vi "Periodic Tasks.vi"(8 "error in":errorcluster) -> ()   [LabVIEW 2023]
doc: "This VI runs in parallel to other tasks. It can contain as many user-defined periodic loops as you need. These can carry out PID or other sorts of timed response."
uses:
  <vilib>/Rock Robotics/WPI/Utilities/WPI_GetSetVariantRefNum.vi
  Robot Global Data.vi
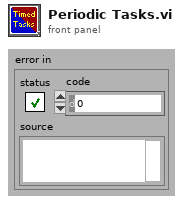
[diagram p1: front panel]
types:
  T1 = typedef "WPI_JoystickDevRef.ctl" = cluster{"Device":T2}
  T2 = typedef "WPI_JoystickDeviceEnum.ctl" = enum16{"USB 0", "USB 1", "USB 2", "USB 3", "USB 4", "USB 5"}
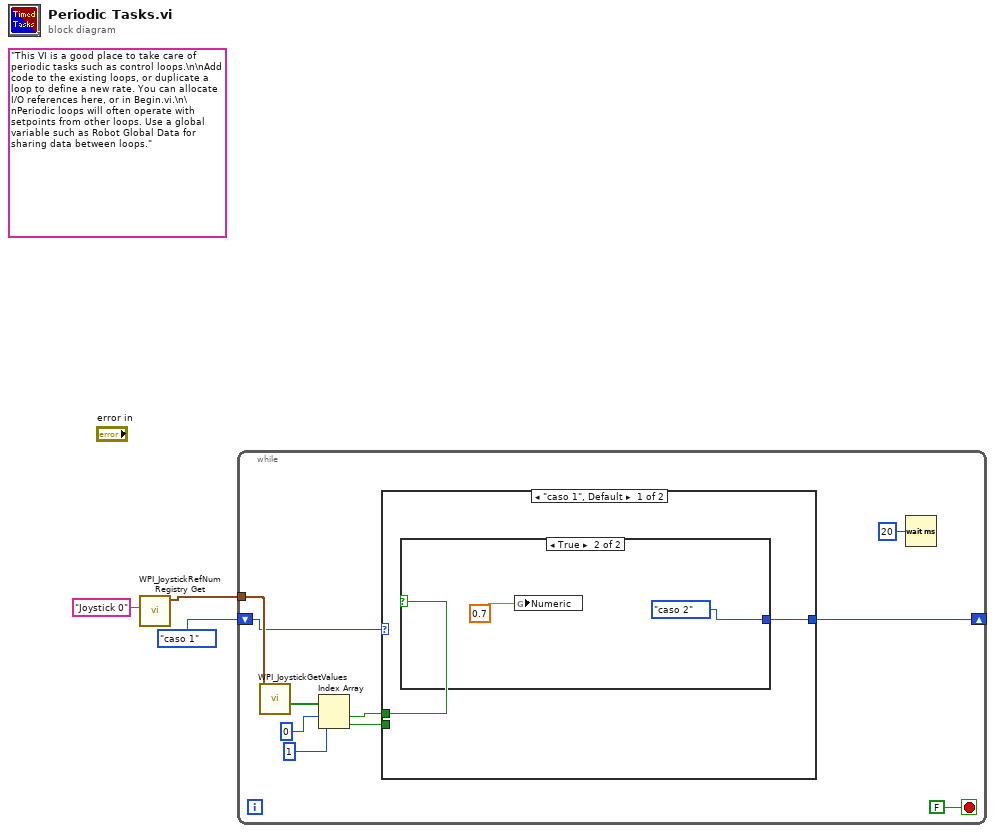
[diagram p0: block diagram]
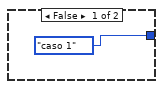
[diagram p2: hidden frame]
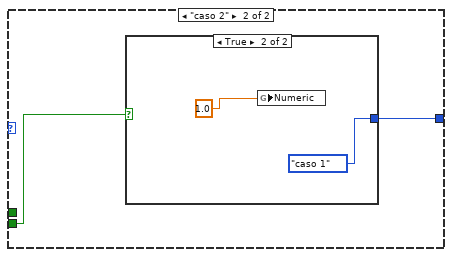
[diagram p3: hidden frame]
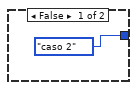
[diagram p4: hidden frame]
diagram:
  (unwired) "This VI is a good place to take care of periodic tasks such as control loops.\n\nAdd code to the existing loops, or duplicate a loop to define a new rate. You can allocate I/O references here, or in Begin.vi.\n\nPeriodic loops will often operate with setpoints from other loops. Use a global variable such as Robot Global Data for sharing data between loops."
  n1 = call <vilib>:"WPI_JoystickRefNum Registry Get.vi"("refnum name"="Joystick 0") -> ("JoystickDevRef"=w2:T1)  [unwired: 9 in, 1 out]
  n2 = while {
    tunnel: w2 -> [w12]
    shift-right: [w5] -> _
    shift-left: enum16{"caso 1", "caso 2"}."caso 1" -> [w8]
    stop <- FALSE stop-if-true
    n3 = call <vilib>:"WPI_JoystickGetValues.vi"("JoystickDevRef"=w12) -> ("Buttons"=w11:bool[])  [unwired: 6 in, 4 out]
    n4 = Index Array(array=w11, index #1=0 ("index"), index #2=1 ("index")) -> (element #1=w7:bool, element #2=w6:bool)
    n5 = case shown="\"caso 1\", Default" w8 {
      tunnel: w7 -> [w15 _]
      tunnel: w6 -> [_ w20]
      tunnel: [w14 w19] -> w5
      frame "caso 1", Default {
        n6 = case shown="True" w15 {
          tunnel: [enum16{"caso 1", "caso 2"}."caso 1" enum16{"caso 1", "caso 2"}."caso 2"] -> w14
          frame False {
          }
          frame True {
            n7 = global write "Robot Global Data.vi" "Numeric"(0.7) -> ()
          }
        }
      }
      frame "caso 2" {
        n8 = case shown="True" w20 {
          tunnel: [enum16{"caso 1", "caso 2"}."caso 2" enum16{"caso 1", "caso 2"}."caso 1"] -> w19
          frame False {
          }
          frame True {
            n9 = global write "Robot Global Data.vi" "Numeric"(1.0) -> ()
          }
        }
      }
    }
    n10 = Wait (ms)(milliseconds to wait=u32 20) -> ()  [unwired: 1 out]
  }
